vi "Latch_RisingEdge.vi"(1 "reset":bool, 2 "set":bool) -> (0 "latch":bool)   [LabVIEW 2014]
panel:
  # "Boolian latch"
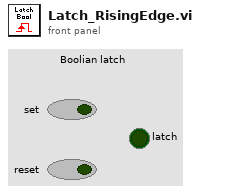
[diagram p1: front panel]
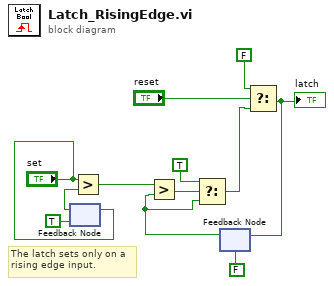
[diagram p0: block diagram]
diagram:
  # "The latch sets only on a\nrising edge input."
  n1 = feedback #1(TRUE ("set")) -> (w3:bool)
  n2 = feedback-in #1("set") -> ()
  n3 = Greater?(x="set", y=w3) -> (0:w4:bool)
  n4 = feedback #2(FALSE ("latch")) -> (w6:bool)
  n5 = Greater?(x=w4, y=w6) -> (0:w10:bool)
  n6 = Select(t=TRUE ("latch"), s=w10, f=w6) -> (s? t:f=w8:bool)
  n7 = Select(t=FALSE ("latch"), s="reset", f=w8) -> (s? t:f=w7:bool)
  "latch" <- w7
  n8 = feedback-in #2(w7) -> ()
